vi "MCCwritevoltage.vi"(2 "error in":errorcluster, 3 "output voltage":dbl=1.0 min=0.0 max=4.0 step=0.5, 4 "task in":refnum<k24>) -> (0 "error out":errorcluster, 1 "task out":refnum<k24>)   [LabVIEW 2012]
uses:
  C:/Program Files (x86)/National Instruments/LabVIEW 2012/vi.lib/ULx/ULx_LV.dll
  Program Files (x86)/National Instruments/LabVIEW 2012/vi.lib/ULx/ULx_LV.dll
  <vilib>/ULx/Write.llb/ULx Write (Analog 1D DBL 1Chan 1Samp).vi
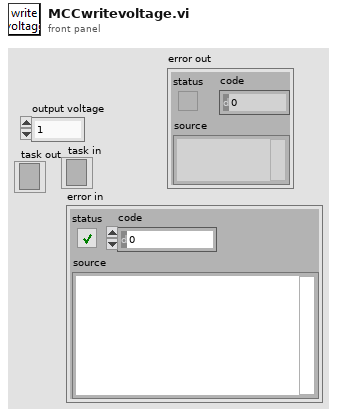
[diagram p1: front panel]
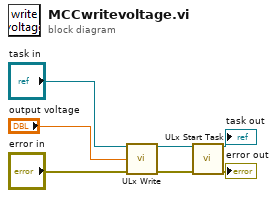
[diagram p0: block diagram]
diagram:
  n1 = call-poly <vilib>:"ULx Write.vi"("task in"="task in", "data"="output voltage", "error in"="error in") -> ("task out"=w2:refnum<k24>, "error out"=w1:errorcluster)  [unwired: 10 in, 1 out]
  n2 = call <vilib>:"ULx Start Task.vi"("task in"=w2, "error in"=w1) -> ("task out"=→"task out":refnum<k24>, "error out"=→"error out":errorcluster)  [unwired: 12 in]
